vi "TDMS Express Write Data (Time Domain).vi"() -> ()   [LabVIEW 2023]
doc: "This example demonstrates how to write time-domain data to a TDMS file using the Write to Measurement File Express VI."
uses:
  Instance           1 47Saved   TDMS - Express write data (time domain) .vi
  Instance           2 47Saved   TDMS - Express write data (time domain) .vi
panel:
  in  "Stop":bool
  out "Waveform Graph":dynamicdata(graph)
  # "Overview: Demonstrates how to write time-domain data to a TDMS file using the Write to Measurement File Express VI.\nInstructions:\n1. Run the VI.\n2. Click Stop to stop the VI."
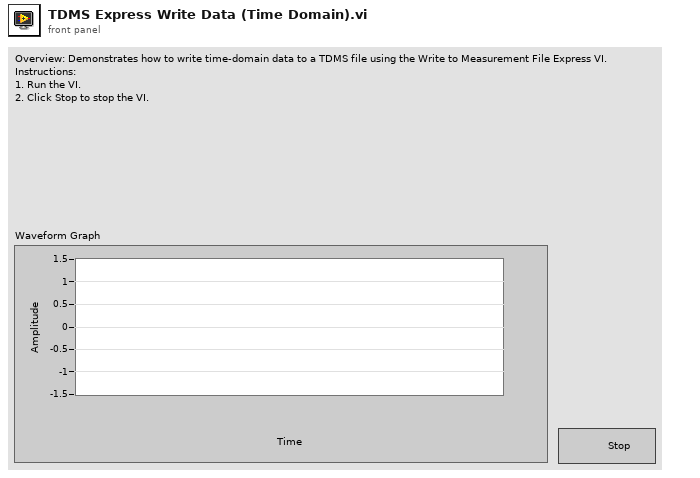
[diagram p1: front panel]
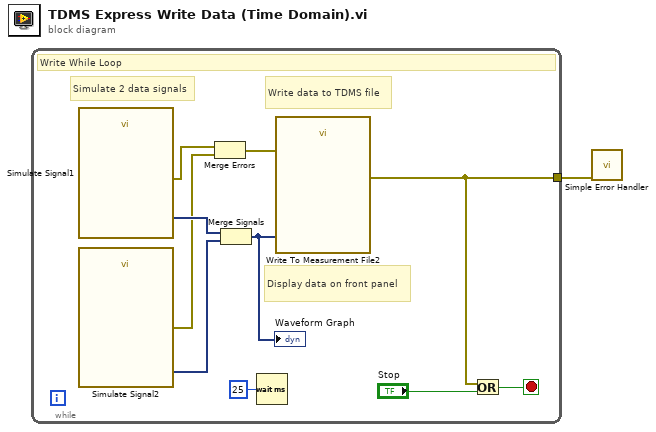
[diagram p0: block diagram]
diagram:
  n1 = while {
    tunnel: [w4] -> w1
    stop <- w2 stop-if-true
    # "Display data on front panel"
    # "Write data to TDMS file"
    # "Simulate 2 data signals"
    # "Write While Loop"
    n2 = call "Simulate Signal1"() -> ("Sine with Uniform Noise"=w11:dynamicdata, "error out"=w7:errorcluster)  [unwired: 8 in, 6 out]
    n3 = call "Simulate Signal2"() -> ("Square with Uniform Noise"=w9:dynamicdata, "error out"=w5:errorcluster)  [unwired: 9 in, 5 out]
    n4 = Merge Errors(w7, w5) -> (w6:errorcluster)
    n5 = Merge Signals(w11, w9) -> (w10:dynamicdata)
    "Waveform Graph" <- w10
    n6 = Wait (ms)(milliseconds to wait=u32 25) -> ()  [unwired: 1 out]
    n7 = call "Write To Measurement File2"("Signals"=w10, "error in (no error)"=w6) -> ("error out"=w4:errorcluster)  [unwired: 15 in, 2 out]
    n8 = Or(x=w4, y="Stop") -> (x .or. y?=w2:bool)
  }
  n9 = call <vilib>:"Simple Error Handler.vi"("error in (no error)"=w1) -> ()  [unwired: 4 in, 5 out]
